vi "ActorDB-VerifyEmptyCluster.vi"(0 "Cluster In":T1) -> (1 "Don't Run Update":bool)   [LabVIEW 2013, in "PartCertDatabase-Actor.lvclass"]
uses:
  PartCertDatabase-Actor.lvclass
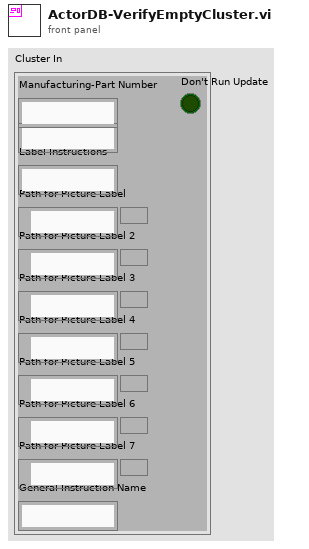
[diagram p1: front panel]
types:
  T1 = cluster{"Manufacturing-Part Number":string, string, "Label Instructions":string, "Path for Picture Label":path, "Path for Picture Label 2":path, "Path for Picture Label 3":path, "Path for Picture Label 4":path, "Path for Picture Label 5":path, "Path for Picture Label 6":path, "Path for Picture Label 7":path, "General Instruction Name":string}
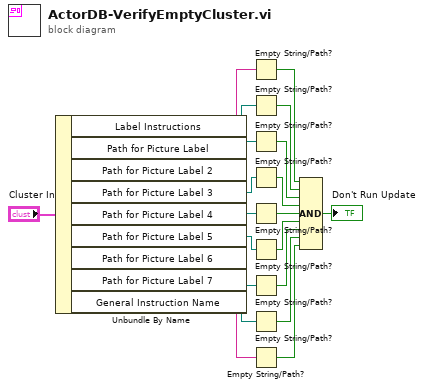
[diagram p0: block diagram]
diagram:
  n1 = Unbundle By Name("Cluster In") -> ("Label Instructions"=w19:string, "Path for Picture Label"=w18:path, "Path for Picture Label 2"=w17:path, "Path for Picture Label 3"=w16:path, "Path for Picture Label 4"=w15:path, "Path for Picture Label 5"=w14:path, "Path for Picture Label 6"=w13:path, "Path for Picture Label 7"=w12:path, "General Instruction Name"=w11:string)
  n2 = Empty String/Path?(string/path=w19) -> (empty?=w10:bool)
  n3 = Empty String/Path?(string/path=w18) -> (empty?=w9:bool)
  n4 = Empty String/Path?(string/path=w17) -> (empty?=w8:bool)
  n5 = Empty String/Path?(string/path=w16) -> (empty?=w7:bool)
  n6 = Empty String/Path?(string/path=w15) -> (empty?=w6:bool)
  n7 = Empty String/Path?(string/path=w14) -> (empty?=w5:bool)
  n8 = Empty String/Path?(string/path=w13) -> (empty?=w4:bool)
  n9 = Empty String/Path?(string/path=w12) -> (empty?=w3:bool)
  n10 = Empty String/Path?(string/path=w11) -> (empty?=w2:bool)
  n11 = Compound Arithmetic op=AND(w10, w9, w8, w7, w6, w5, w4, w3, w2) -> (→"Don't Run Update":bool)
